vi "DeserializeInitTargetObjectAndStack.vi"(4 "Preservation Options":T2, 6 "expand objects on type conflict?":bool, 8 "error in (no error)":errorcluster, 9 "ClassName Cache":refnum<data-value>, 10 "Wired object (not default)":refnum<class>, 11 "From object (default value)":refnum<class>) -> (0 "error out":errorcluster, 1 "NumLevelsExpanded":u16, 2 "Object stack (child, parent)":T1[](array[typedef]), 3 "Target Object":refnum<class "BlueSerializable.lvclass">)   [LabVIEW 2020, in "BlueSerialization.lvlib" / "BlueSerializer.lvclass"]
uses:
  BlueSerializer.lvclass
  BlueSerializer.lvclass/BlueSerializer.ctl
  BlueSerializable/BlueSerializable.lvclass
  DeserializePreservationOptions.ctl
  ClassNameObj.ctl
  ClassNameCacheMap.ctl
  Support/SetSerializableDataObject.ctl
  PreserveNonWiredDataOption.ctl
  ClassNameCacheCluster.ctl
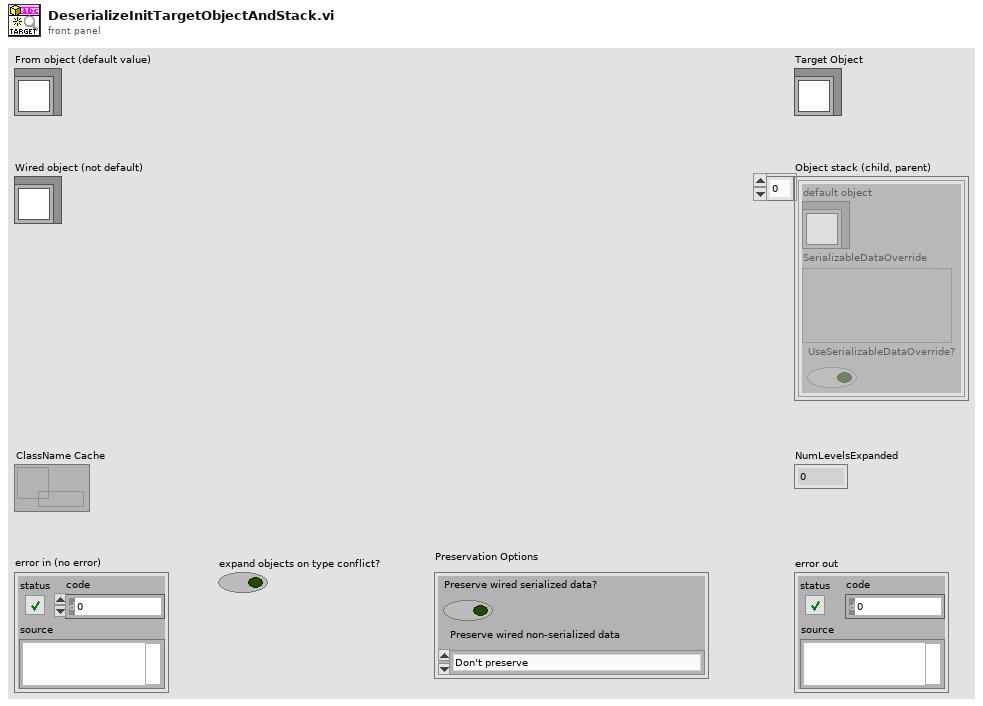
[diagram p1: front panel]
types:
  T1 = typedef "BlueSerialization.lvlib/BlueSerializer.lvclass/SetSerializableDataObject.ctl" = cluster{"default object":refnum<class "BlueSerializable.lvclass">, "SerializableDataOverride":variant, "UseSerializableDataOverride?":bool}
  T2 = typedef "BlueSerialization.lvlib/BlueSerializer.lvclass/DeserializePreservationOptions.ctl" = cluster{"Preserve wired serialized data?":bool, "Preserve wired non-serialized data":T3}
  T3 = typedef "BlueSerialization.lvlib/BlueSerializer.lvclass/PreserveNonWiredDataOption.ctl" = enum16{"Don't preserve", "Preserve (error on less-specific wired types)", "Preserve (except on less-specific wired types)"}
  T4 = typedef "BlueSerialization.lvlib/BlueSerializer.lvclass/ClassNameSummary.ctl" = enum16{"sibling", "more specific", "less specific", "same"}
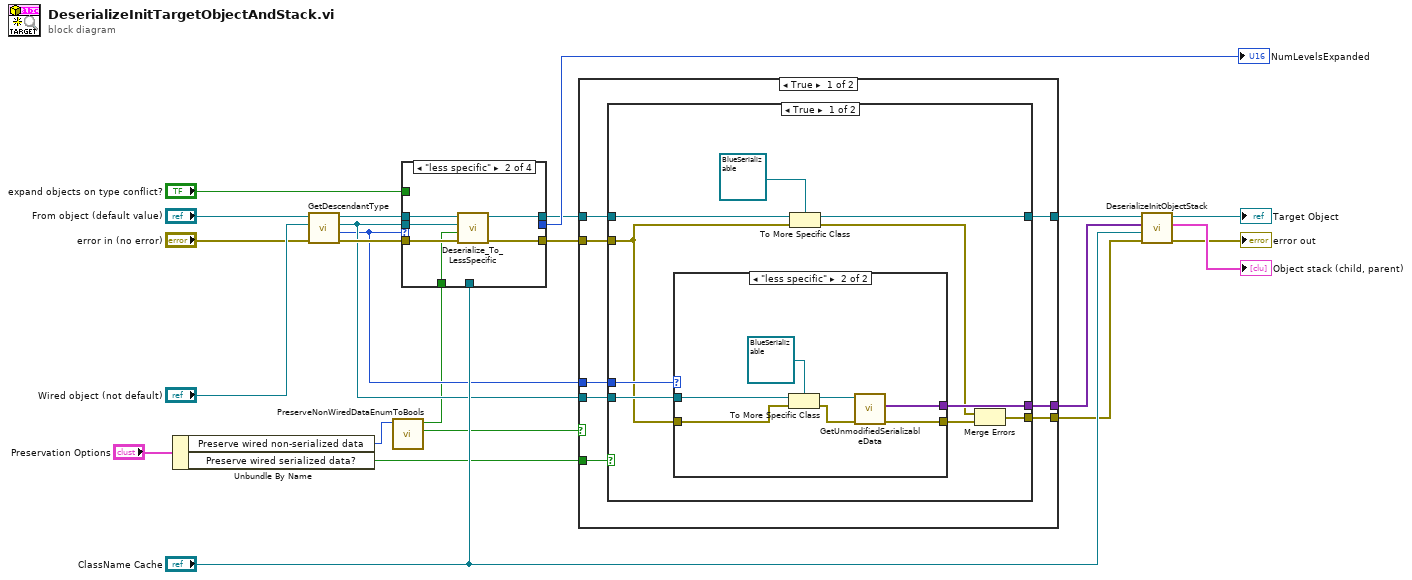
[diagram p0: block diagram]
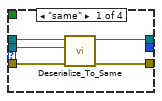
[diagram p2: hidden frame]
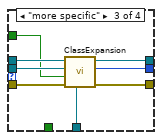
[diagram p3: hidden frame]
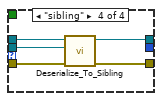
[diagram p4: hidden frame]
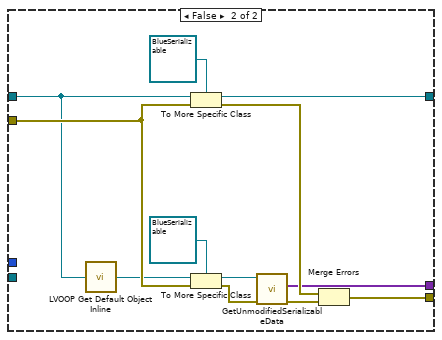
[diagram p6: hidden frame]
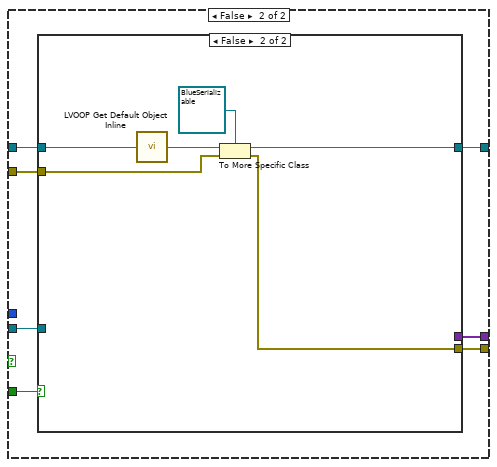
[diagram p7: hidden frame]
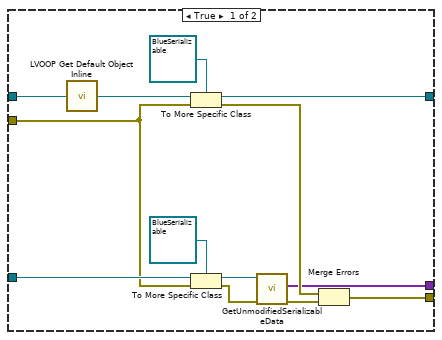
[diagram p8: hidden frame]
diagram:
  n1 = Unbundle By Name("Preservation Options") -> ("Preserve wired non-serialized data"=w3:T3, "Preserve wired serialized data?"=w14:bool)
  n2 = call "GetDescendantType.vi"("error in (no error)"="error in (no error)", "To Object"="Wired object (not default)", "From Object"="From object (default value)") -> ("error out"=w9:errorcluster, "Descent Type"=w6:T4, "To Object (dup)"=w7:refnum<class>, "From Object (dup)"=w10:refnum<class>)  [unwired: 5 in]
  n3 = call "PreserveNonWiredDataEnumToBools.vi"("Preserve wired non-serialized data"=w3) -> ("Preserve wired non-serialized data?"=w2:bool, "Error on less-specific wired types?"=w1:bool)  [unwired: 9 in]
  n4 = case shown="\"less specific\"" w6 {
    tunnel: w10 -> [w28 w34 w42 w47]
    tunnel: w7 -> [w27 w33 w41 w46]
    tunnel: w9 -> [w26 w32 w38 w45]
    tunnel: [w25 w30 w39 w44] -> w8
    tunnel: "expand objects on type conflict?" -> [_ _ w40 _]
    tunnel: [w24 w31 w37 w43] -> w4
    tunnel: [_ _ w36 _] -> w15
    tunnel: "ClassName Cache" -> [_ _ w35 _]
    tunnel: w1 -> [_ w29 _ _]
    frame "same" {
      n5 = call "Deserialize_To_Same.vi"("error in (no error)"=w26, "To Object"=w27, "From Object"=w28) -> ("error out"=w24:errorcluster, "Target Object"=w25:refnum<class>)  [unwired: 7 in]
    }
    frame "less specific" {
      n6 = call "Deserialize_To_LessSpecific.vi"("error in (no error)"=w32, "Error on less-specific wired types?"=w29, "To Object"=w33, "From Object"=w34) -> ("error out"=w31:errorcluster, "Target Object"=w30:refnum<class>)  [unwired: 6 in]
    }
    frame "more specific" {
      n7 = call "ClassExpansion.vi"("ClassName Cache"=w35, "error in (no error)"=w38, "expand objects on type conflict?"=w40, "To Object"=w41, "From Object"=w42) -> ("error out"=w37:errorcluster, "NumLevelsExpanded"=w36:u16, "Target object"=w39:refnum<class>)  [unwired: 4 in]
    }
    frame "sibling" {
      n8 = call "Deserialize_To_Sibling.vi"("error in (no error)"=w45, "To Object"=w46, "From Object"=w47) -> ("error out"=w43:errorcluster, "Target Object"=w44:refnum<class>)  [unwired: 7 in]
    }
  }
  "NumLevelsExpanded" <- w15
  n9 = case shown="True" w2 {
    tunnel: w14 -> [w55 w92]
    tunnel: w8 -> [w54 w91]
    tunnel: [w53 w90] -> w13
    tunnel: [w52 w89] -> w12
    tunnel: [w51 w88] -> w11
    tunnel: w7 -> [w49 w87]
    tunnel: w6 -> [w50 _]
    tunnel: w4 -> [w48 w86]
    frame True {
      n10 = case shown="True" w55 {
        tunnel: w54 -> [w64 w75]
        tunnel: [w63 w80] -> w53
        tunnel: [w58 w77] -> w52
        tunnel: [w60 w76] -> w51
        tunnel: w50 -> [w61 _]
        tunnel: w49 -> [w62 _]
        tunnel: w48 -> [w56 w85]
        frame True {
          n11 = case shown="\"less specific\"" w61 {
            tunnel: [_ w68] -> w60
            tunnel: [w66 w70] -> w59
            tunnel: w62 -> [_ w69]
            tunnel: w56 -> [w66 w67]
            frame "sibling", "more specific", "same" {
              # "No need to override.\nTarget object has the data!\n(This is an optimization)"
            }
            frame "less specific" {
              n12 = To More Specific Class(target class=refnum<class "BlueSerializable.lvclass"> refnum ("BlueSerializer.lvlib:BlueSerializable.lvclass"), reference=w69, error in=w67) -> (specific class reference=w73:refnum<class "BlueSerializable.lvclass">, error out=w72:errorcluster)
              n13 = call "GetUnmodifiedSerializableData.vi"("error in (no error)"=w72, "BlueSerializable in"=w73) -> ("error out"=w70:errorcluster, "SerializableData (parent,child)"=w68:variant[])  [unwired: 7 in, 1 out]
            }
          }
          n14 = To More Specific Class(target class=refnum<class "BlueSerializable.lvclass"> refnum ("BlueSerializer.lvlib:BlueSerializable.lvclass"), reference=w64, error in=w56) -> (specific class reference=w63:refnum<class "BlueSerializable.lvclass">, error out=w57:errorcluster)
          n15 = Merge Errors(w57, w59) -> (w58:errorcluster)
        }
        frame False {
          n16 = call "LVOOP Get Default Object Inline.vi"("Object"=w75) -> ("Object Default Instance"=w74:refnum<class>)
          n17 = To More Specific Class(target class=refnum<class "BlueSerializable.lvclass"> refnum ("BlueSerializer.lvlib:BlueSerializable.lvclass"), reference=w75, error in=w85) -> (specific class reference=w80:refnum<class "BlueSerializable.lvclass">, error out=w79:errorcluster)
          n18 = To More Specific Class(target class=refnum<class "BlueSerializable.lvclass"> refnum ("BlueSerializer.lvlib:BlueSerializable.lvclass"), reference=w74, error in=w85) -> (specific class reference=w82:refnum<class "BlueSerializable.lvclass">, error out=w83:errorcluster)
          n19 = call "GetUnmodifiedSerializableData.vi"("error in (no error)"=w83, "BlueSerializable in"=w82) -> ("error out"=w78:errorcluster, "SerializableData (parent,child)"=w76:variant[])  [unwired: 7 in, 1 out]
          n20 = Merge Errors(w79, w78) -> (w77:errorcluster)
        }
      }
    }
    frame False {
      n21 = case shown="False" w92 {
        tunnel: w91 -> [w94 w107]
        tunnel: [w99 w110] -> w90
        tunnel: [w98 w109] -> w89
        tunnel: [w97 _] -> w88
        tunnel: w87 -> [w96 _]
        tunnel: w86 -> [w95 w108]
        frame True {
          n22 = call "LVOOP Get Default Object Inline.vi"("Object"=w94) -> ("Object Default Instance"=w93:refnum<class>)
          n23 = To More Specific Class(target class=refnum<class "BlueSerializable.lvclass"> refnum ("BlueSerializer.lvlib:BlueSerializable.lvclass"), reference=w93, error in=w95) -> (specific class reference=w99:refnum<class "BlueSerializable.lvclass">, error out=w102:errorcluster)
          n24 = To More Specific Class(target class=refnum<class "BlueSerializable.lvclass"> refnum ("BlueSerializer.lvlib:BlueSerializable.lvclass"), reference=w96, error in=w95) -> (specific class reference=w103:refnum<class "BlueSerializable.lvclass">, error out=w104:errorcluster)
          n25 = call "GetUnmodifiedSerializableData.vi"("error in (no error)"=w104, "BlueSerializable in"=w103) -> ("error out"=w101:errorcluster, "SerializableData (parent,child)"=w97:variant[])  [unwired: 7 in, 1 out]
          n26 = Merge Errors(w102, w101) -> (w98:errorcluster)
        }
        frame False {
          n27 = call "LVOOP Get Default Object Inline.vi"("Object"=w107) -> ("Object Default Instance"=w106:refnum<class>)
          n28 = To More Specific Class(target class=refnum<class "BlueSerializable.lvclass"> refnum ("BlueSerializer.lvlib:BlueSerializable.lvclass"), reference=w106, error in=w108) -> (specific class reference=w110:refnum<class "BlueSerializable.lvclass">, error out=w109:errorcluster)
        }
      }
    }
  }
  n29 = call "DeserializeInitObjectStack.vi"("error in (no error)"=w12, "ClassName Cache"="ClassName Cache", "SerializableDataOverride (parent, child)"=w11, "Target Object"=w13) -> ("error out"=→"error out":errorcluster, "Object stack (child, parent)"=→"Object stack (child, parent)":T1[], "Target Object (dup)"=→"Target Object":refnum<class "BlueSerializable.lvclass">)  [unwired: 5 in]
